vi "User Interface Global.vi"(6 "data2":variant, 7 "command (Update UI)":T2=enum."Update UI", 8 "error in":errorcluster, 9 "data1":variant, 10 "action":T1, 11 "user interface queue reference":T3) -> (0 "error out":errorcluster)   [LabVIEW 2011]
uses:
  Controls/User Interface Queue Reference.ctl
  Controls/User Interface Control.ctl
  Controls/User Interface Action.ctl
  User Interface Global Action.ctl
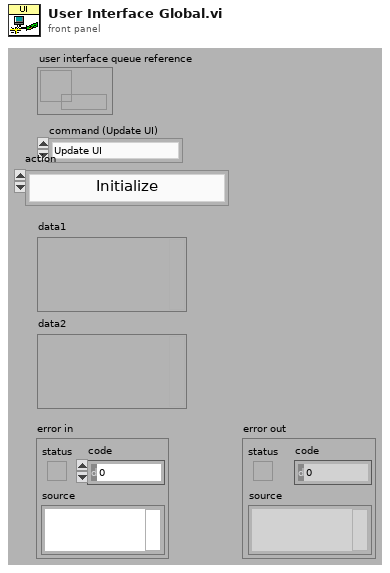
[diagram p1: front panel]
types:
  T1 = typedef "User Interface Action.ctl" = enum16{"Initialize", "Update Real Channel", "Update Imag Channel", "Update Re/Im channel @ Hardware Ctrl", "Pulse Sequence", "Visibility Front Panel Controls", "Report Custom Errors", "Set Pulse Sequence Type", "Update Pulse Timings", "Update Transfer Time", "Update Status Bar", "Set Sequence Progress", "Set 90 Degree Pulse Sequence Params", "Set CMPG Pulse Sequence Parms", "Set T1 Pulse Sequence Params", "Stop"}
  T2 = typedef "User Interface Global Action.ctl" = enum16{"Initialize", "Update UI", "Stop"}
  T3 = typedef "User Interface Queue Reference.ctl" = refnum<queue>
  T4 = typedef "User Interface Control.ctl" = cluster{"data1":variant, "data2":variant, "action":T1}
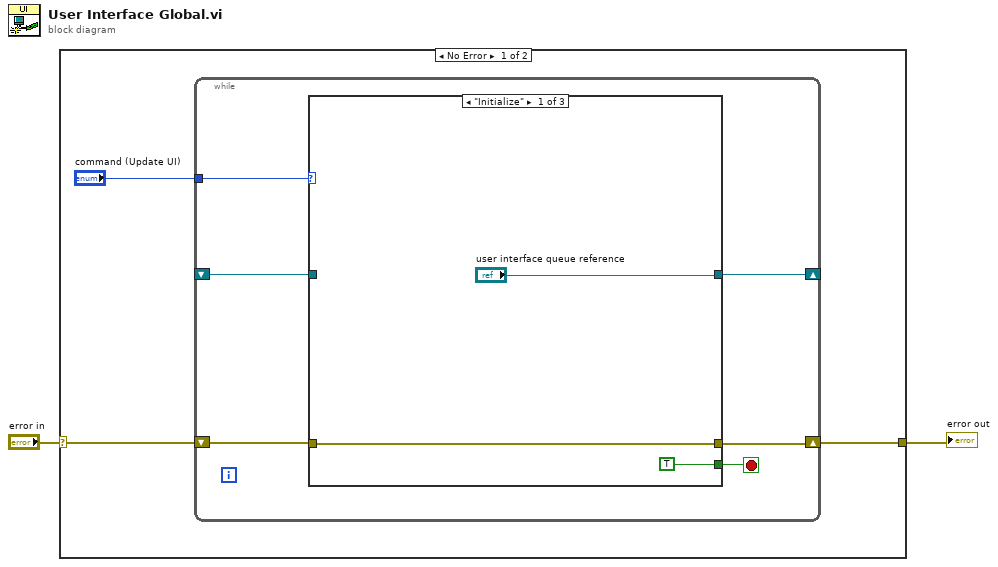
[diagram p0: block diagram]
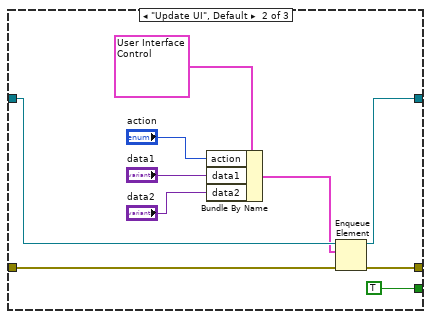
[diagram p2: hidden frame]
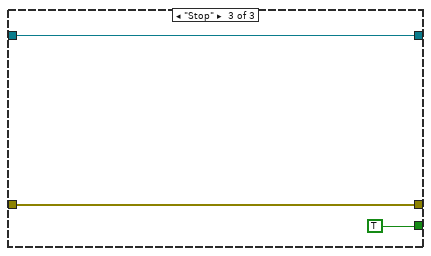
[diagram p3: hidden frame]
diagram:
  n1 = case shown="No Error" "error in" {
    selector: "error in" -> [w5 w28]
    tunnel: [w4 w28] -> w1
    frame No Error {
      n2 = while {
        shift-right: [w9] -> w4
        shift-left: w5 -> [w10]
        tunnel: "command (Update UI)" -> [w8]
        shift-right: [w7] -> _
        shift-left: _ -> [w6]
        stop <- w11 stop-if-true
        n3 = case shown="\"Initialize\"" w8 {
          tunnel: [TRUE TRUE TRUE] -> w11
          tunnel: w10 -> [w13 w22 w27]
          tunnel: [w13 w21 w27] -> w9
          tunnel: ["user interface queue reference" w19 w25] -> w7
          tunnel: w6 -> [_ w20 w25]
          frame "Initialize" {
          }
          frame "Update UI", Default {
            n4 = Bundle By Name(cluster=T4 {"data1"=variant, "data2"=variant, "action"=enum."Initialize"} ("GUI control"), "action"="action", "data1"="data1", "data2"="data2") -> (w15:T4)
            n5 = Enqueue Element(queue=w20, element=w15, error in (no error)=w22) -> (queue out=w19:T3, error out=w21:errorcluster)  [unwired: 1 in, 1 out]
          }
          frame "Stop" {
          }
        }
      }
    }
    frame Error {
    }
  }
  "error out" <- w1
